vi "XML Read Tag.vi"(10 "XML":string="<math resultRef=\"-2\"><ml:eval><ml:id xml:space=\"preserve\"><Span xmlns=\"http://schemas.microsoft.com/winfx/2006/xaml/presentation\" xmlns:pw=\"clr-namespace:Ptc.Wpf;assembly=Ptc.Core\">N<pw:Subscript>SedTanks</pw:Subscript></Span></ml:id><ml:result /></ml:eval></math>", 11 "XML Tag":string="region") -> (1 "Found":bool, 2 "content":string, 3 "tag parameter":string)   [LabVIEW 2011, in "Design Server.lvlib"]
uses:
  Design Server.lvlib
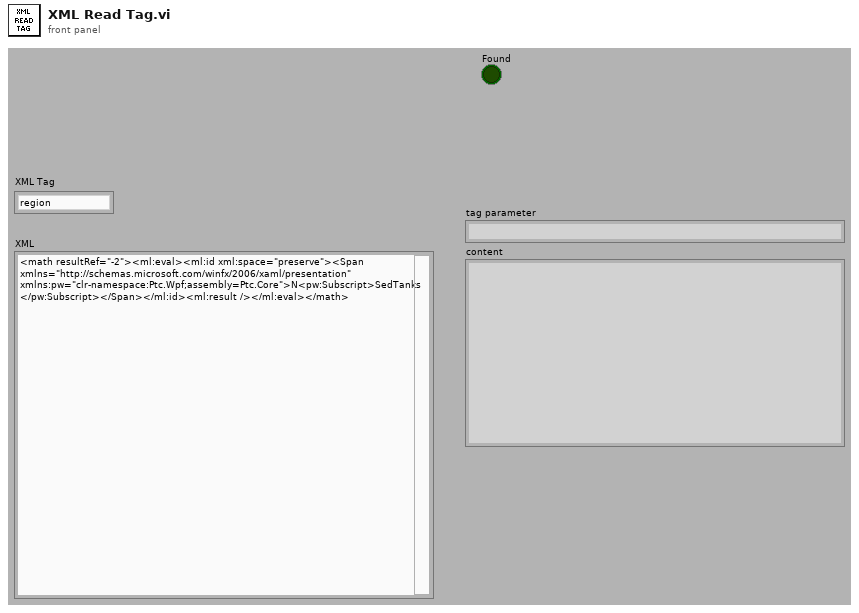
[diagram p1: front panel]
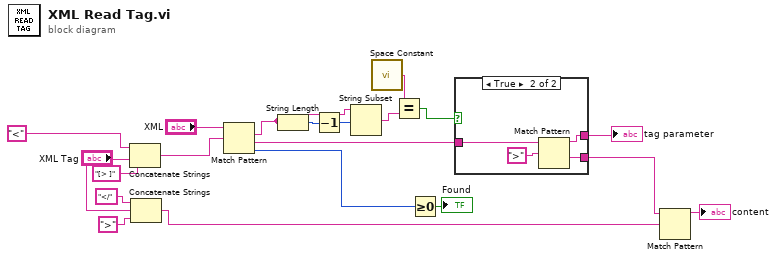
[diagram p0: block diagram]
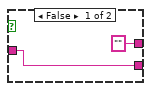
[diagram p2: hidden frame]
diagram:
  n1 = Concatenate Strings("<" ("string"), "XML Tag", "[> ]" ("string")) -> (w19:string)
  n2 = Concatenate Strings("</" ("string"), "XML Tag", ">" ("regular expression")) -> (w15:string)
  n3 = Match Pattern(string="XML", regular expression=w19) -> (match substring=w1:string, after substring=w13:string, offset past match=w9:i32)  [unwired: 1 in, 1 out]
  n4 = String Length(string=w1) -> (length=w6:i32)
  n5 = Decrement(x=w6) -> (x-1=w2:i32)
  n6 = String Subset(string=w1, offset (0)=w2) -> (substring=w5:string)  [unwired: 1 in]
  n7 = call <vilib>:"Space Constant.vi"() -> ("String"=w4:string)
  n8 = Equal?(x=w4, y=w5) -> (x = y?=w3:bool)
  n9 = Greater Or Equal To 0?(x=w9) -> (x >= 0?=→"Found":bool)
  n10 = case shown="True" w3 {
    tunnel: w13 -> [w22 w26]
    tunnel: [w22 w24] -> w12
    tunnel: ["" ("XML") w23] -> w11
    frame False {
    }
    frame True {
      n11 = Match Pattern(string=w26, regular expression=">") -> (before substring=w23:string, after substring=w24:string)  [unwired: 1 in, 2 out]
    }
  }
  "tag parameter" <- w11
  n12 = Match Pattern(string=w12, regular expression=w15) -> (before substring=→"content":string)  [unwired: 1 in, 3 out]
